vi "Get Variant Data.vi"(8 "error in (no error)":errorcluster, 11 "Data in":string) -> (0 "error out":errorcluster, 2 "Variant":variant, 3 "Data out":string)   [LabVIEW 2013, in "Hierarchy Framework.lvlib" / "Section.lvclass"]
uses:
  Section.lvclass
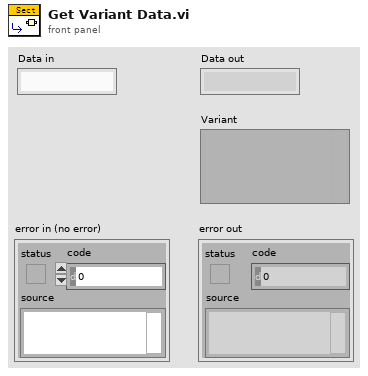
[diagram p1: front panel]
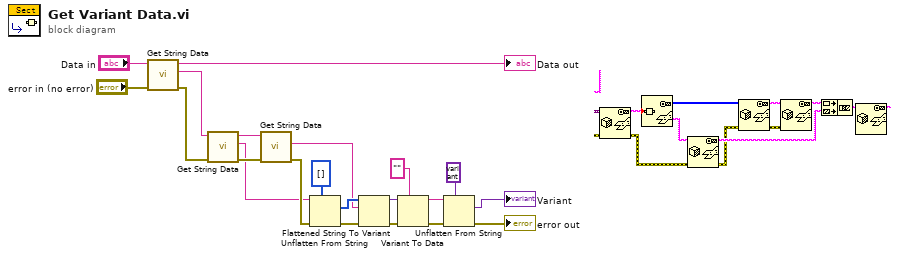
[diagram p0: block diagram]
diagram:
  n1 = call "Get String Data.vi"("error in (no error)"="error in (no error)", "Data in"="Data in") -> ("error out"=w20:errorcluster, "String"=w18:string, "Data out"=→"Data out":string)  [unwired: 7 in]
  n2 = call "Get String Data.vi"("error in (no error)"=w20, "Data in"=w18) -> ("error out"=w16:errorcluster, "String"=w15:string, "Data out"=w17:string)  [unwired: 7 in]
  n3 = call "Get String Data.vi"("error in (no error)"=w16, "Data in"=w17) -> ("error out"=w19:errorcluster, "String"=w12:string)  [unwired: 7 in, 1 out]
  n4 = Unflatten From String(type=i16[] [] ("类型字符串"), binary string=w15, error in (no error)=w19) -> (value=w13:i16[], error out=w21:errorcluster)  [unwired: 2 in, 1 out]
  n5 = Flattened String To Variant(4:w21, 6:w12, 7:w13) -> (0:w7:errorcluster, 3:w8:variant)
  n6 = Variant To Data(error in=w7, type="" ("String"), Variant=w8) -> (data=w4:string, error out=w5:errorcluster)
  n7 = Unflatten From String(type=variant ("变体"), binary string=w4, error in (no error)=w5) -> (value=→"Variant":variant, error out=→"error out":errorcluster)  [unwired: 2 in, 1 out]
